vi "Place Orders.vi"(8 "error in (no error)":errorcluster, 10 "Items":refnum<class "Beverage.lvclass">[](array[class]), 11 "Cashier in":refnum<class "Cashier.lvclass">) -> (0 "error out":errorcluster, 3 "Cashier out":refnum<class "Cashier.lvclass">)   [LabVIEW 2020, in "Cashier.lvclass"]
uses:
  Cashier.lvclass
  Support/Beverages/Beverage/Beverage.lvclass
  C:/Users/anton/Documents/GitHub/Triarc-Examples/Coffee Shop/Worker/Worker.lvclass
  Worker/Worker.lvclass/Worker.ctl
  Process Job/Job Handler.lvclass
  Worker/Worker.lvclass
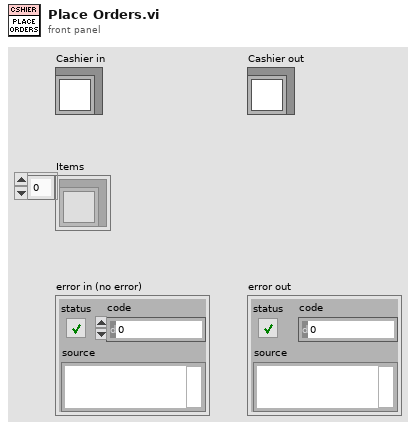
[diagram p1: front panel]
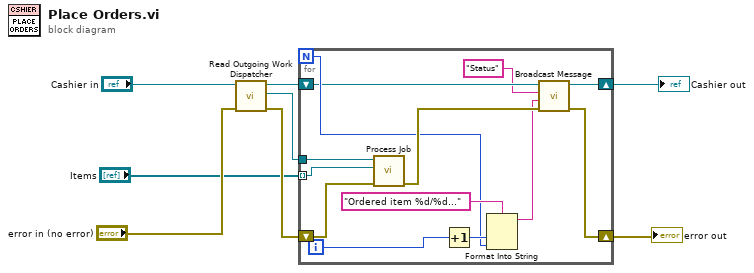
[diagram p0: block diagram]
diagram:
  n1 = call "Read Outgoing Work Dispatcher.vi"("error in (no error)"="error in (no error)", "Worker In"="Cashier in") -> ("error out"=w8:errorcluster, "Job Handler"=w4:refnum<class "Job Handler.lvclass">, "Worker Out"=w2:refnum<class "Cashier.lvclass">)  [unwired: 7 in]
  n2 = for {
    N -> [w14]
    tunnel: w4 -> [w21]
    tunnel: "Items" -> [w20] mode=indexing
    shift-right: [w13] -> w6
    shift-left: w8 -> [w19]
    shift-right: [w11] -> w1
    shift-left: w2 -> [w12]
    i -> [w16]
    n3 = call-dynamic "Process Job.vi"("error in (no error)"=w19, "Task"=w20, "Process Job In"=w21) -> ("error out"=w18:errorcluster)  [unwired: 7 in, 1 out]
    n4 = Increment(x=w16) -> (x+1=w17:i32)
    n5 = Format Into String(format string="Ordered item %d/%d..." ("Ordered Item"), w17, w14) -> (resulting string=w10:string)  [unwired: 2 in, 1 out]
    n6 = call-dynamic "Broadcast Message.vi"("error in (no error)"=w18, "Message Data"=w10, "Message"="Status", "Rig Process In"=w12) -> ("error out"=w13:errorcluster, "Rig Process Out"=w11:refnum<class "Cashier.lvclass">)  [unwired: 6 in]
  }
  "error out" <- w6
  "Cashier out" <- w1
